vi "TTA_MATLAB_Run_System.vi"(11 "error in":errorcluster) -> (15 "error out":errorcluster)   [LabVIEW 2016]
uses:
  TTA_Globals/Test_Environment.vi
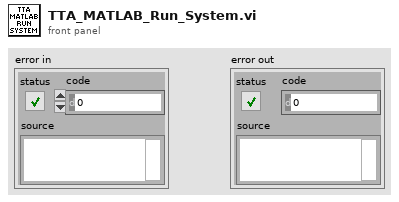
[diagram p1: front panel]
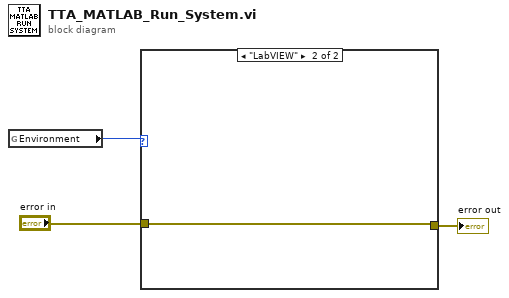
[diagram p0: block diagram]
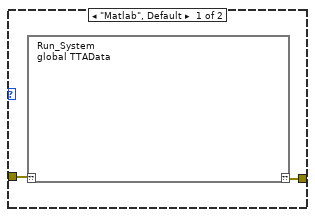
[diagram p2: hidden frame]
diagram:
  n1 = global read "Test_Environment.vi" "Environment"() -> (w1:enum16{"Matlab", "LabVIEW"})
  n2 = case shown="\"LabVIEW\"" w1 {
    tunnel: "error in" -> [w5 w6]
    tunnel: [w4 w6] -> w2
    frame "Matlab", Default {
      n3 = script code="Run_System\nglobal TTAData"("??"=w5) -> ("??"=w4:errorcluster)
    }
    frame "LabVIEW" {
    }
  }
  "error out" <- w2
